vi "Right Front Panel (SubVI).vi"() -> ()   [LabVIEW 2015]
uses:
  Left Variables.vi
panel:
  in  "STOP":bool
  out "L Tilt Count":i32
  out "Heading":dbl
  out "Center X":dbl
  out "Center Y":dbl
  out "rc X":dbl
  out "rc Y":dbl
  out "lc X":dbl
  out "lc Y":dbl
  out "L Avg LB Y Center":dbl
  out "L Avg RB X Center":dbl
  out "L Avg RB Y Center":dbl
  out "L Avg LB X Center":dbl
  out "L Average Distance (ft)":dbl
  out "L Distance (ft)":dbl
  out "L Pan Angle":dbl
  out "L Raw RB Y Center":u16
  out "L Raw RB X Center":u16
  out "L Raw LB Y Center":u16
  out "L Raw LB X Center":u16
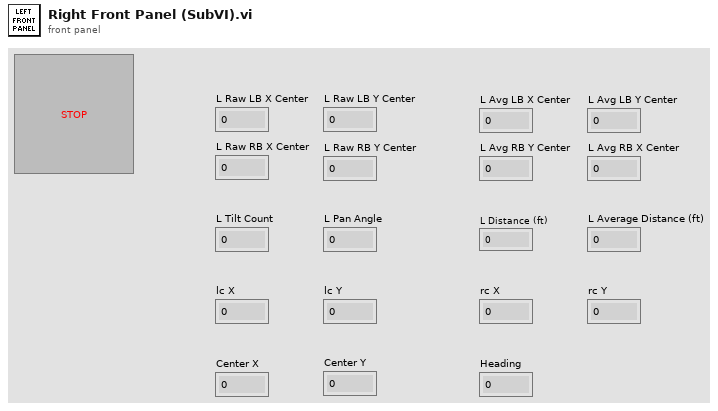
[diagram p1: front panel]
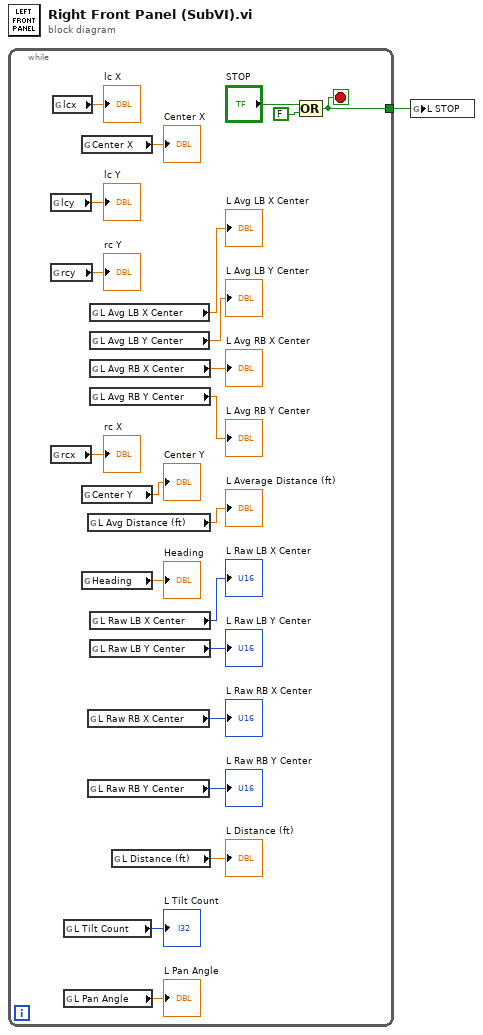
[diagram p0: block diagram]
diagram:
  n1 = while {
    tunnel: [w2] -> w1
    stop <- w2 stop-if-true
    n2 = global read "Left Variables.vi" "lcy"() -> (→"lc Y":dbl)
    n3 = global read "Left Variables.vi" "rcy"() -> (→"rc Y":dbl)
    n4 = global read "Left Variables.vi" "rcx"() -> (→"rc X":dbl)
    n5 = global read "Left Variables.vi" "lcx"() -> (→"lc X":dbl)
    n6 = global read "Left Variables.vi" "L Tilt Count"() -> (→"L Tilt Count":i32)
    n7 = global read "Left Variables.vi" "L Pan Angle"() -> (→"L Pan Angle":dbl)
    n8 = global read "Left Variables.vi" "Center X"() -> (→"Center X":dbl)
    n9 = global read "Left Variables.vi" "Center Y"() -> (→"Center Y":dbl)
    n10 = global read "Left Variables.vi" "Heading"() -> (→"Heading":dbl)
    n11 = global read "Left Variables.vi" "L Avg Distance (ft)"() -> (→"L Average Distance (ft)":dbl)
    n12 = global read "Left Variables.vi" "L Raw RB X Center"() -> (→"L Raw RB X Center":u16)
    n13 = global read "Left Variables.vi" "L Raw RB Y Center"() -> (→"L Raw RB Y Center":u16)
    n14 = global read "Left Variables.vi" "L Avg LB X Center"() -> (→"L Avg LB X Center":dbl)
    n15 = global read "Left Variables.vi" "L Avg LB Y Center"() -> (→"L Avg LB Y Center":dbl)
    n16 = global read "Left Variables.vi" "L Avg RB X Center"() -> (→"L Avg RB X Center":dbl)
    n17 = global read "Left Variables.vi" "L Avg RB Y Center"() -> (→"L Avg RB Y Center":dbl)
    n18 = global read "Left Variables.vi" "L Raw LB X Center"() -> (→"L Raw LB X Center":u16)
    n19 = global read "Left Variables.vi" "L Raw LB Y Center"() -> (→"L Raw LB Y Center":u16)
    n20 = global read "Left Variables.vi" "L Distance (ft)"() -> (→"L Distance (ft)":dbl)
    n21 = Compound Arithmetic op=OR("STOP", FALSE ("y")) -> (w2:bool)
  }
  n22 = global write "Left Variables.vi" "L STOP"(w1) -> ()
